vi "Empty VArray Constant.vi"() -> (0 "Empty Cluster":variant)   [LabVIEW 2020, in "openg_variant.lvlib"]
uses:
  openg_variant.lvlib
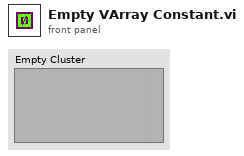
[diagram p1: front panel]
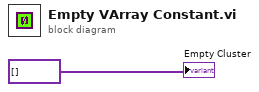
[diagram p0: block diagram]
diagram:
  "Empty Cluster" <- variant[] [] ("Array")
